vi "test convert complex to bytestring.vi"() -> ()   [LabVIEW 2018, in "LV-Julia_ZMQ-Roundtrip_lib.lvlib"]
uses:
  LV-Julia_ZMQ-Roundtrip_lib.lvlib
  d9e6895c-6e91-421e-b7c0-309ac06110dd.vi
  d9e6895c-6e91-421e-b7c0-309ac06110dd.vi/c2df5bd4-805a-4ea3-81db-5efb946f76d3.vi
  d9e6895c-6e91-421e-b7c0-309ac06110dd.vi/c2df5bd4-805a-4ea3-81db-5efb946f76d3.vi/72a641be-d6f4-46d9-845c-556ad676036c.vi
  d9e6895c-6e91-421e-b7c0-309ac06110dd.vi/c2df5bd4-805a-4ea3-81db-5efb946f76d3.vi/72a641be-d6f4-46d9-845c-556ad676036c.vi/12c26963-c1bc-4536-9660-69e03f0fe55c.vi
  check ID validity.vi
panel:
  in  "data in":csg=2.0+0.0i
  out "unsigned byte array":u8[](array[numeric])=[0, 0, 0, 64, 0, 0, 0, 0]
  out "bindata":u8[](array[numeric])=[0, 0, 0, 0, 0, 0, 0, 64]
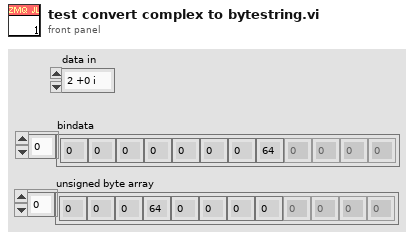
[diagram p1: front panel]
types:
  T1 = enum16{"big-endian, network order", "native, host order", "little-endian"}
  T2 = typedef "Bindata&description.ctl" = cluster{"bindata_descr":T3[], "bindata":u8[]}
  T3 = typedef "LV-Julia_ZMQ-Roundtrip_lib.lvlib/Bindata description.ctl" = cluster{"nofbytes":i32, "numtype":string, "start":i32, "arrdims":i32[], "kwarg_name":string, "category":string}
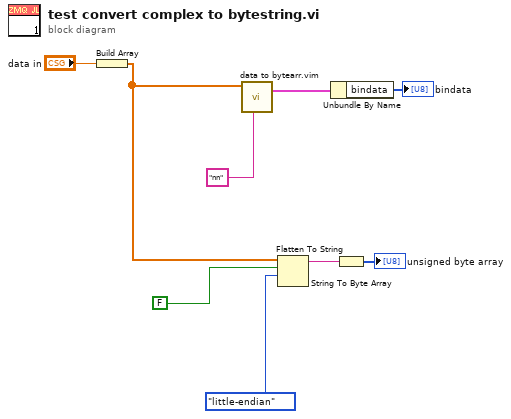
[diagram p0: block diagram]
diagram:
  n1 = Build Array("data in") -> (w1:csg[])
  n2 = call "data to bytearr.vim"("kwarg_name"="nn", "data in"=w1) -> ("Bindata & descr out"=w8:T2)  [unwired: 7 in, 2 out]
  n3 = Flatten To String(anything=w1, prepend array or string size? (T)=FALSE, byte order (0:big-endian, network order)=T1."little-endian" ("byte order")) -> (data string=w5:string)  [unwired: 1 in, 2 out]
  n4 = Unbundle By Name(w8) -> ("bindata"=→"bindata":u8[])
  n5 = String To Byte Array(string=w5) -> (unsigned byte array=→"unsigned byte array":u8[])
